vi "Key - MCListbox Write.vi"(4 "write raw string? (F)":bool, 6 "Remove \\r\\n":bool, 7 "delimiter (,)":string=",", 8 "error in (no error)":errorcluster, 10 "MulticolumnListbox Ref in":refnum<vi>, 11 "refnum":T1) -> (0 "error out":errorcluster, 2 "size(s)":i32[](array[numeric]), 3 "Refnum out":T1, 5 "Column Header Strings[]":string[](array[string]))   [LabVIEW 2013]
uses:
  <vilib>/Utility/config.llb/Config Data RefNum.ctl
  <vilib>/Utility/config.llb/Write Key (String).vi
  <vilib>/Utility/config.llb/NI_LVConfig.lvlib
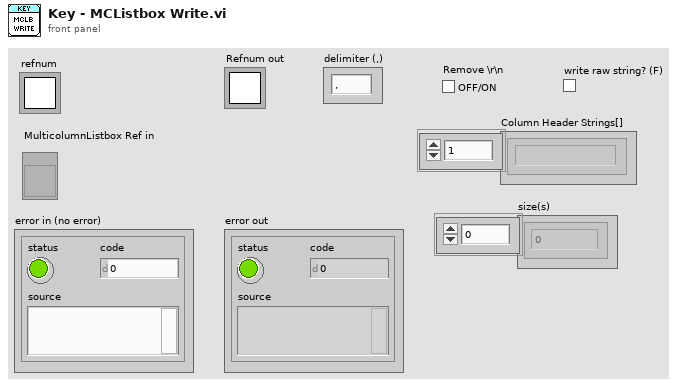
[diagram p1: front panel]
types:
  T1 = typedef "NI_LVConfig.lvlib/Config Data RefNum.ctl" = refnum<k1>
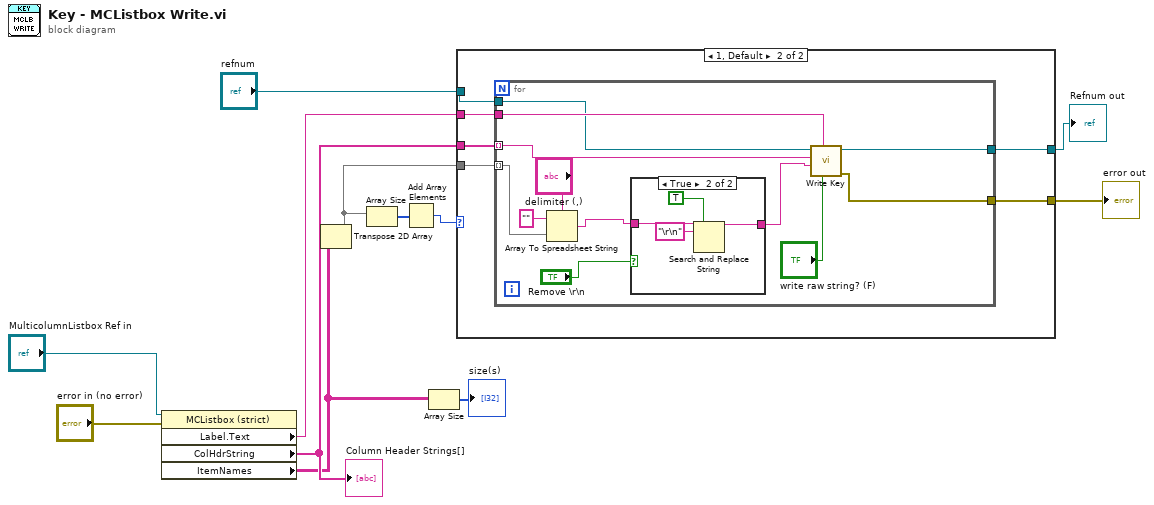
[diagram p0: block diagram]
diagram:
  n1 = property on="Property Node" class="MCListbox (strict)"(reference="MulticolumnListbox Ref in", error in="error in (no error)") -> ("Label.Text"=w9:string, "ColHdrString"=w10:string[], "ItemNames"=w5:string[][])  [unwired: 2 out]
  "Column Header Strings[]" <- w10
  n2 = Transpose 2D Array(2D array=w5) -> (transposed array=w3:string[][])
  n3 = Array Size(array=w3) -> (size(s)=w1:i32[])
  n4 = Add Array Elements(numeric array=w1) -> (sum=w2:i32)
  n5 = Array Size(array=w5) -> (size(s)=→"size(s)":i32[])
  n6 = case shown="1, Default" w2 {
    tunnel: w10 -> [_ w19]
    tunnel: w9 -> [_ w18]
    tunnel: "refnum" -> [w13 w17]
    tunnel: [w13 w16] -> w7
    tunnel: [_ w15] -> w6
    tunnel: w3 -> [_ w14]
    frame 0 {
    }
    frame 1, Default {
      n7 = for {
        tunnel: w19 -> [w31] mode=indexing
        tunnel: w14 -> [w27] mode=indexing
        tunnel: w18 -> [w30]
        tunnel: w17 -> [w26]
        tunnel: [w25] -> w16
        tunnel: [w24] -> w15
        n8 = Array To Spreadsheet String(delimiter (Tab)="delimiter (,)", array=w27, 3:"" ("format string")) -> (spreadsheet string=w22:string)
        n9 = case shown="True" "Remove \\r\\n" {
          tunnel: w22 -> [w32 w36]
          tunnel: [w32 w33] -> w21
          frame False {
          }
          frame True {
            n10 = Search and Replace String(replace all?=TRUE ("replace all? (F)"), input string=w36, search string="\r\n") -> (result string=w33:string)  [unwired: 5 in, 3 out]
          }
        }
        n11 = call-poly <vilib>:"Write Key.vi"("write raw string? (F)"="write raw string? (F)", "section"=w30, "value"=w21, "key"=w31, "refnum"=w26) -> ("error out"=w24:errorcluster, "refnum out"=w25:T1)  [unwired: 4 in, 1 out]
      }
    }
  }
  "Refnum out" <- w7
  "error out" <- w6
